vi "Follower Setter.vi"(0 "DeviceReference":T1, 3 "Update Frequency (Hz)":dbl=100.0, 5 "StopSendingOtherRequests":bool=TRUE, 7 "MasterID":i32, 9 "OpposeMasterDirection":bool) -> (4 "DeviceReference Out":T1)   [LabVIEW 2023]
doc: "Follow the motor output of another Talon.\nIf Talon is in torque control, the torque is copied - which will increase the total torque applied. If Talon is in percent supply output control, the duty cycle is matched. Motor direction either matches master's configured direction or opposes it based on OpposeMasterDirection."
uses:
  Users/Cory/Documents/PhoenixPro-LabVIEW-Generation/controls/DeviceReference.ctl
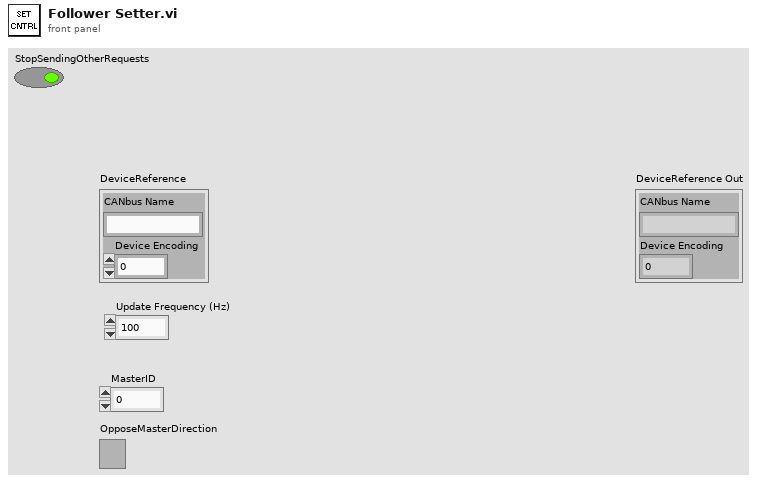
[diagram p1: front panel]
types:
  T1 = typedef "DeviceReference.ctl" = cluster{"CANbus Name":string, "Device Encoding":u32}
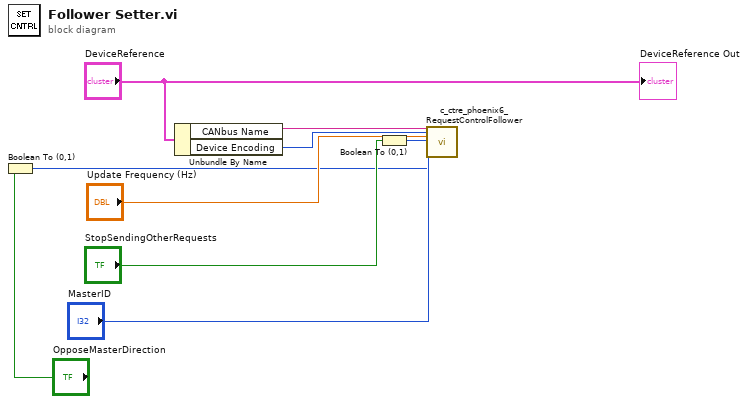
[diagram p0: block diagram]
diagram:
  n1 = Boolean To (0,1)(Boolean="OpposeMasterDirection") -> (0, 1=w1:i16)
  n2 = Unbundle By Name("DeviceReference") -> ("CANbus Name"=w8:string, "Device Encoding"=w7:u32)
  n3 = Boolean To (0,1)(Boolean="StopSendingOtherRequests") -> (0, 1=w4:i16)
  n4 = call <vilib>:"c_ctre_phoenix6_RequestControlFollower.vi"("String"=w8, "Numeric 2"=w7, "Numeric 3"="Update Frequency (Hz)", "Numeric 4"=w4, "Numeric 5"="MasterID", "Numeric 6"=w1) -> ()  [unwired: 21 in, 1 out]
  "DeviceReference Out" <- "DeviceReference"
